vi "Supply_ReadCurrent.vi"(8 "error in (no error)":errorcluster, 11 "SupplyControl in":refnum<class "SupplyControl.lvclass">) -> (0 "error out":errorcluster, 2 "Current in nA":dbl format="%#.6g", 3 "SupplyControl out":refnum<class "SupplyControl.lvclass">)   [LabVIEW 2013, in "SupplyControl.lvclass"]
uses:
  SupplyControl.lvclass
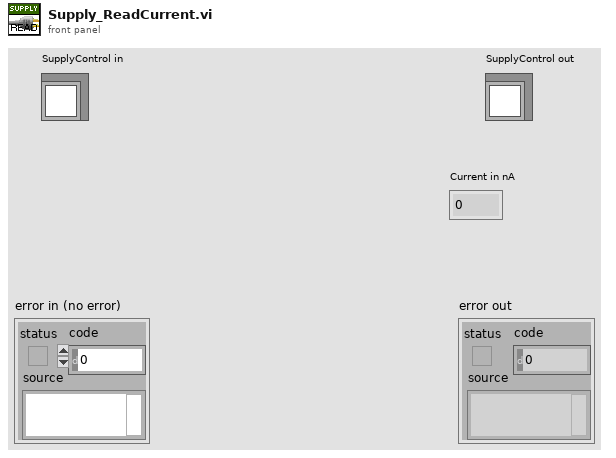
[diagram p1: front panel]
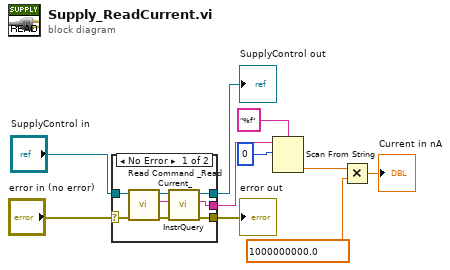
[diagram p0: block diagram]
diagram:
  n1 = case shown="No Error" "error in (no error)" {
    selector: "error in (no error)" -> [w11 w19]
    tunnel: [w18 w19] -> w7
    tunnel: [w17 w20] -> w8
    tunnel: "SupplyControl in" -> [w13 w20]
    tunnel: [w12 _] -> w3
    frame No Error {
      n2 = call-dynamic "Read Command _Read Current_.vi"("error in (no error)"=w11, "SupplyControl in"=w13) -> ("error out"=w16:errorcluster, "Command \"Read Current\""=w15:string, "SupplyControl out"=w14:refnum<class "SupplyControl.lvclass">)  [unwired: 7 in]
      n3 = call-dynamic "InstrQuery.vi"("error in (no error)"=w16, "Command string"=w15, "InstControl in"=w14) -> ("error out"=w18:errorcluster, "Instrument response"=w12:string, "InstControl out"=w17:refnum<class "SupplyControl.lvclass">)  [unwired: 6 in]
    }
    frame Error {
    }
  }
  "SupplyControl out" <- w8
  "error out" <- w7
  n4 = Scan From String(format string="%f", input string=w3, initial scan location=0) -> (output 1=w5:dbl)  [unwired: 2 in, 3 out]
  n5 = Multiply(x=w5, y=1000000000.0) -> (x*y=→"Current in nA":dbl)
